vi "AE75TX Read.vi"(7 "Scaling Coefficients":T1, 8 "error in":errorcluster, 10 "Modbus Configuration":T8, 11 "Modbus Master in":refnum<class "Modbus Master.lvclass">) -> (0 "error out":errorcluster, 1 "DER_Measurement":T2, 2 "DER_Status":T4, 3 "Modbus Master out":refnum<class "Modbus Master.lvclass">, 4 "IED_Status":T6)   [LabVIEW 2018, in "AE75TX Actor.lvlib" / "AE75TX.lvclass"]
uses:
  AE75TX.lvclass
  <vilib>/Modbus/master/Modbus Master.lvclass
  Controls/Modbus Configuration Cluster.ctl
  <vilib>/ORNL/CSEISMIC DDS/CSEISMIC DDS Base/Data Types/Controls/DeviceID.ctl
  <vilib>/ORNL/CSEISMIC DDS/CSEISMIC DDS Base/Data Types/IED_Status.ctl
  <vilib>/ORNL/CSEISMIC DDS/CSEISMIC DDS Base/Data Types/Controls/Timestamp.ctl
  <vilib>/ORNL/CSEISMIC DDS/CSEISMIC DDS Base/Data Types/DER_Status.ctl
  <vilib>/ORNL/CSEISMIC DDS/CSEISMIC DDS Base/Data Types/Controls/DroopCurve.ctl
  <vilib>/ORNL/CSEISMIC DDS/CSEISMIC DDS Base/Data Types/DER_Measurement.ctl
  Controls/Scaling Coefficients Measurements.ctl
  Controls/PV Standard Value Cluster.ctl
  <vilib>/ORNL/CSEISMIC DDS/CSEISMIC DDS Base/CSEISMIC DDS.lvclass
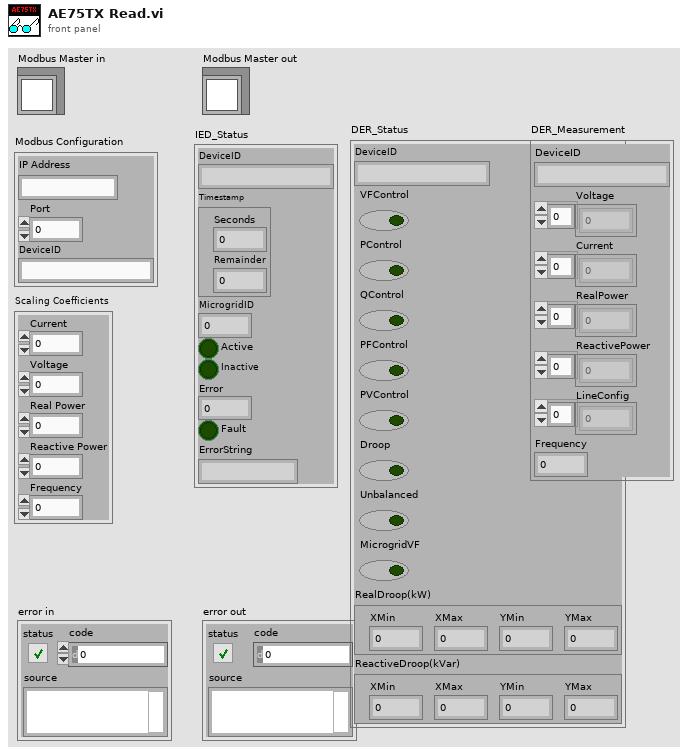
[diagram p1: front panel]
types:
  T1 = typedef "AE75TX Actor.lvlib/AE75TX.lvclass/Scaling Coefficients Measurements.ctl" = cluster{"Current":dbl, "Voltage":dbl, "Real Power":dbl, "Reactive Power":dbl, "Frequency":dbl}
  T2 = typedef "CSEISMIC DDS.lvlib/CSEISMIC DDS.lvclass/DER_Measurement.ctl" = cluster{"DeviceID":T3, "Voltage":dbl[], "Current":dbl[], "RealPower":dbl[], "ReactivePower":dbl[], "LineConfig":u8[], "Frequency":dbl}
  T3 = typedef "CSEISMIC DDS.lvlib/CSEISMIC DDS.lvclass/DeviceID.ctl" = string
  T4 = typedef "CSEISMIC DDS.lvlib/CSEISMIC DDS.lvclass/DER_Status.ctl" = cluster{"DeviceID":T3, "VFControl":bool, "PControl":bool, "QControl":bool, "PFControl":bool, "PVControl":bool, "Droop":bool, "Unbalanced":bool, "MicrogridVF":bool, "RealDroop(kW)":T5, "ReactiveDroop(kVar)":T5}
  T5 = typedef "CSEISMIC DDS.lvlib/CSEISMIC DDS.lvclass/DroopCurve.ctl" = cluster{"XMin":dbl, "XMax":dbl, "YMin":dbl, "YMax":dbl}
  T6 = typedef "CSEISMIC DDS.lvlib/CSEISMIC DDS.lvclass/IED_Status.ctl" = cluster{"DeviceID":T3, "Timestamp":T7, "MicrogridID":u8, "Active":bool, "Inactive":bool, "Error":i32, "Fault":bool, "ErrorString":string}
  T7 = typedef "CSEISMIC DDS.lvlib/CSEISMIC DDS.lvclass/Timestamp.ctl" = cluster{"Seconds":u64, "Remainder":u64}
  T8 = typedef "AE75TX Actor.lvlib/AE75TX.lvclass/Modbus Configuration Cluster.ctl" = cluster{"IP Address":string, "Port":u16, "DeviceID":T3}
  T9 = typedef "AE75TX Actor.lvlib/AE75TX.lvclass/PV Standard Value Cluster.ctl" = cluster{"Va (V)":sgl, "Vb (V)":sgl, "Vc (V)":sgl, "Ia (A)":sgl, "Ib (A)":sgl, "Ic (A)":sgl, "Vdc (V)":sgl, "Idc (A)":sgl, "Frequency (Hz)":sgl, "Line Power (kW)":sgl, "Total Power (kWh)":u32, "PV Input (V)":sgl, "DC Power (kW)":sgl}
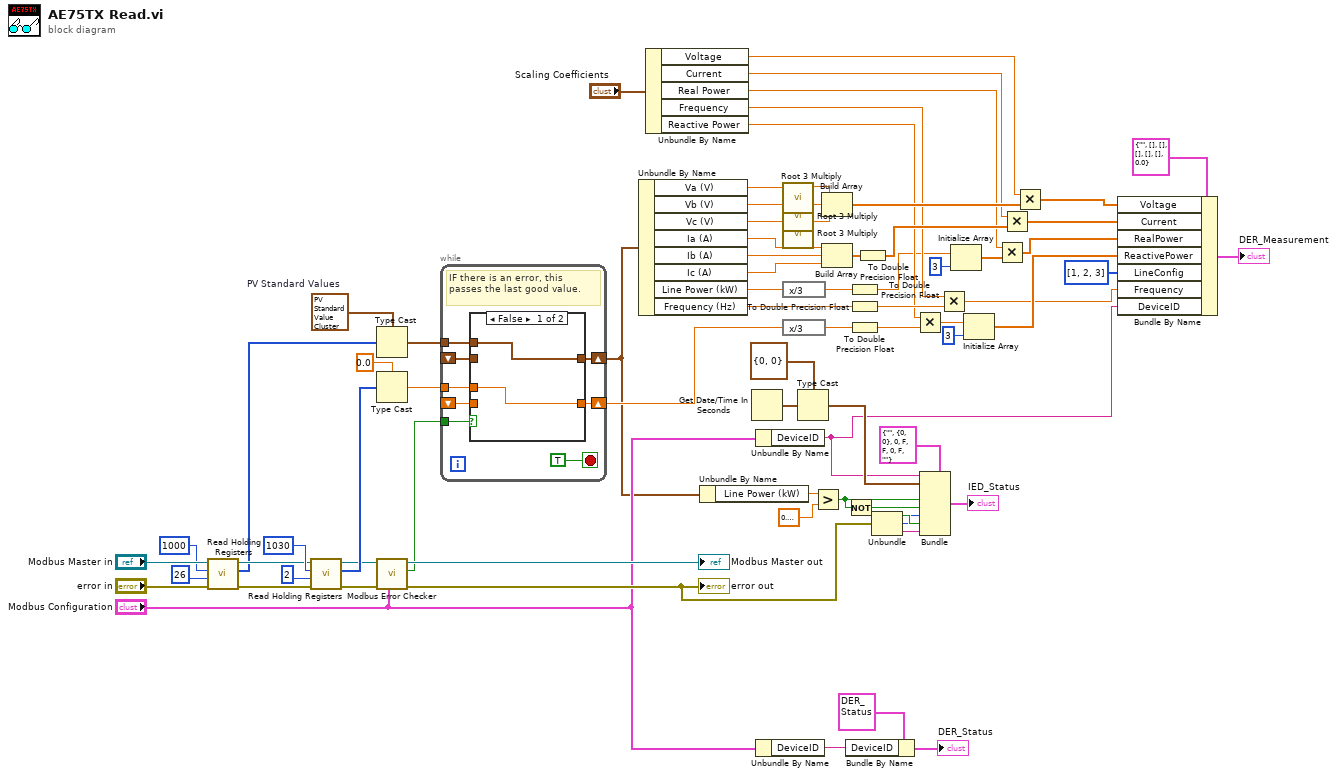
[diagram p0: block diagram]
diagram:
  w65 = T9 {"Va (V)"=0.0, "Vb (V)"=0.0, "Vc (V)"=0.0, "Ia (A)"=0.0, "Ib (A)"=0.0, "Ic (A)"=0.0, "Vdc (V)"=0.0, "Idc (A)"=0.0, "Frequency (Hz)"=0.0, "Line Power (kW)"=0.0, "Total Power (kWh)"=0, "PV Input (V)"=0.0, "DC Power (kW)"=0.0}  # PV Standard Values
  n1 = call-dynamic "Read Holding Registers.vi"("error in (no error)"="error in", "number of holding registers"=u16 26, "starting address"=u16 1000, "Modbus master in"="Modbus Master in") -> ("error out"=w71:errorcluster, "register values"=w64:u16[], "Modbus master out"=w70:refnum<class "Modbus Master.lvclass">)  [unwired: 5 in]
  n2 = call-dynamic "Read Holding Registers.vi"("error in (no error)"=w71, "number of holding registers"=u16 2, "starting address"=u16 1030, "Modbus master in"=w70) -> ("error out"=w63:errorcluster, "register values"=w74:u16[], "Modbus master out"=w61:refnum<class "Modbus Master.lvclass">)  [unwired: 5 in]
  n3 = Type Cast(type=w65, x=w64) -> (*(type *) &x=w1:T9)
  n4 = Type Cast(type=sgl 0.0, x=w74) -> (*(type *) &x=w2:sgl)
  n5 = call "Modbus Error Checker.vi"("Modbus Configuration"="Modbus Configuration", "error in"=w63, "Modbus Master in"=w61) -> ("error out"=w55:errorcluster, "Error Handled"=w3:bool, "Modbus Master out"=→"Modbus Master out":refnum<class "Modbus Master.lvclass">)  [unwired: 6 in]
  "error out" <- w55
  n6 = while {
    shift-right: [w81] -> w4
    shift-left: _ -> [w77]
    shift-right: [w79] -> w5
    shift-left: _ -> [w76]
    tunnel: w3 -> [w82]
    tunnel: w2 -> [w78]
    tunnel: w1 -> [w80]
    stop <- TRUE stop-if-true
    # "IF there is an error, this passes the last good value."
    n7 = case shown="False" w82 {
      tunnel: [w85 w87] -> w81
      tunnel: w80 -> [w85 _]
      tunnel: [w84 w86] -> w79
      tunnel: w78 -> [w84 _]
      tunnel: w77 -> [_ w87]
      tunnel: w76 -> [_ w86]
      frame False {
      }
      frame True {
      }
    }
  }
  n8 = Unbundle By Name(w4) -> ("Va (V)"=w41:sgl, "Vb (V)"=w40:sgl, "Vc (V)"=w39:sgl, "Ia (A)"=w35:sgl, "Ib (A)"=w34:sgl, "Ic (A)"=w33:sgl, "Line Power (kW)"=w31:sgl, "Frequency (Hz)"=w20:sgl)
  n9 = Unbundle By Name("Scaling Coefficients") -> ("Voltage"=w28:dbl, "Current"=w25:dbl, "Real Power"=w22:dbl, "Frequency"=w18:dbl, "Reactive Power"=w15:dbl)
  n10 = Unbundle By Name(w4) -> ("Line Power (kW)"=w60:sgl)
  n11 = Get Date/Time In Seconds() -> (seconds since 1Jan1904=w48:timestamp)
  n12 = Unbundle By Name("Modbus Configuration") -> ("DeviceID"=w7:T3)
  n13 = Unbundle By Name("Modbus Configuration") -> ("DeviceID"=w45:T3)
  n14 = call "Root 3 Multiply.vi"("RMS Line to Neutral"=w41) -> ("RMS Line to Line"=w37:dbl)  [unwired: 10 in]
  n15 = call "Root 3 Multiply.vi"("RMS Line to Neutral"=w40) -> ("RMS Line to Line"=w38:dbl)  [unwired: 10 in]
  n16 = call "Root 3 Multiply.vi"("RMS Line to Neutral"=w39) -> ("RMS Line to Line"=w36:dbl)  [unwired: 10 in]
  n17 = expression code="x/3"(w31) -> (w21:sgl)
  n18 = expression code="x/3"(w5) -> (w17:sgl)
  n19 = Type Cast(type=T7 {"Seconds"=0, "Remainder"=0} ("Timestamp"), x=w48) -> (*(type *) &x=w47:T7)
  n20 = Greater?(x=w60, y=sgl 0.1) -> (0:w57:bool)
  n21 = Build Array(w37, w38, w36) -> (w27:dbl[])
  n22 = Build Array(w35, w34, w33) -> (w32:sgl[])
  n23 = Not(x=w57) -> (.not. x?=w56:bool)
  n24 = Bundle By Name(cluster=T4 {"DeviceID"="", "VFControl"=FALSE, "PControl"=FALSE, "QControl"=FALSE, "PFControl"=FALSE, "PVControl"=FALSE, "Droop"=FALSE, "Unbalanced"=FALSE, "MicrogridVF"=FALSE, "RealDroop(kW)"={"XMin"=0.0, "XMax"=0.0, "YMin"=0.0, "YMax"=0.0}, "ReactiveDroop(kVar)"={"XMin"=0.0, "XMax"=0.0, "YMin"=0.0, "YMax"=0.0}} ("DER_Status"), "DeviceID"=w45) -> (→"DER_Status":T4)
  n25 = To Double Precision Float(number=w21) -> (double precision float=w14:dbl)
  n26 = To Double Precision Float(number=w20) -> (double precision float=w19:dbl)
  n27 = To Double Precision Float(number=w17) -> (double precision float=w16:dbl)
  n28 = To Double Precision Float(number=w32) -> (double precision float=w23:dbl[])
  n29 = Unbundle(w55) -> ("status"=w54:bool, "code"=w51:i32, "source"=w53:string)
  n30 = Multiply(x=w15, y=w16) -> (x*y=w9:dbl)
  n31 = Bundle(cluster=T6 {"DeviceID"="", "Timestamp"={"Seconds"=0, "Remainder"=0}, "MicrogridID"=0, "Active"=FALSE, "Inactive"=FALSE, "Error"=0, "Fault"=FALSE, "ErrorString"=""} ("output cluster"), "DeviceID"=w7, "Timestamp"=w47, "Active"=w57, "Inactive"=w56, "Error"=w51, "Fault"=w54, "ErrorString"=w53) -> (→"IED_Status":T6)  [unwired: 1 in]
  n32 = Multiply(x=w18, y=w19) -> (x*y=w6:dbl)
  n33 = Initialize Array(w14, 3 ("dimension size")) -> (w12:dbl[])
  n34 = Initialize Array(w9, 3 ("dimension size")) -> (w8:dbl[])
  n35 = Multiply(x=w22, y=w12) -> (x*y=w11:dbl[])
  n36 = Multiply(x=w25, y=w23) -> (x*y=w24:dbl[])
  n37 = Multiply(x=w28, y=w27) -> (x*y=w26:dbl[])
  n38 = Bundle By Name(cluster=T2 {"DeviceID"="", "Voltage"=[], "Current"=[], "RealPower"=[], "ReactivePower"=[], "LineConfig"=[], "Frequency"=0.0} ("DER_Measurement"), "Voltage"=w26, "Current"=w24, "RealPower"=w11, "ReactivePower"=w8, "LineConfig"=u8[] [1, 2, 3], "Frequency"=w6, "DeviceID"=w7) -> (→"DER_Measurement":T2)
